vi "Init_Instr.vi"(8 "error in (no error)":errorcluster caption="entrée d'erreur (pas d'erreur)", 11 "Class Instrument Multimeter en entrée":refnum<class "Class Instrument Schielding_Box.lvclass">) -> (0 "error out":errorcluster caption="sortie d'erreur", 3 "Class Instrument Multimeter en sortie":refnum<class "Class Instrument Schielding_Box.lvclass">)   [LabVIEW 2020, in "Library Instrument & Equipement.lvlib" / "Library Instruments.lvlib" / "Class Instrument Schielding_Box.lvclass"]
uses:
  Class Instrument Schielding_Box.lvclass
  Instrument (Default)/Class Instrument (Default).lvclass
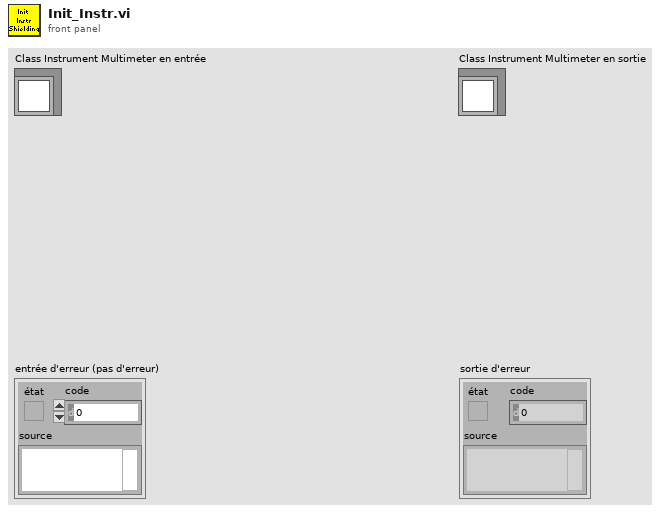
[diagram p1: front panel]
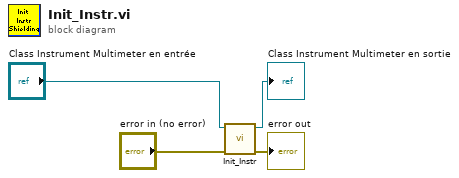
[diagram p0: block diagram]
diagram:
  n1 = call-parent "Init_Instr.vi"("error in (no error)"="error in (no error)", "Class Instrument (Default) en entrée"="Class Instrument Multimeter en entrée") -> ("error out"=→"error out":errorcluster, "Class Instrument (Default) en sortie"=→"Class Instrument Multimeter en sortie":refnum<class "Class Instrument Schielding_Box.lvclass">)  [unwired: 8 in]
